vi "Generate symbol map.vi"(11 "M":i32) -> (3 "symbol map":cdb[](array[numeric]) format="%.3f")   [LabVIEW 2011]
uses:
  <vilib>/Analysis/Matrix/Numeric/Conversions/Array To Matrix - RA2.vi
  <vilib>/addons/Modulation/Digital/General/MT Generate Symbol Map (Rectangular).vi
  <vilib>/addons/Modulation/niDMT.lvlib
  <vilib>/Analysis/Matrix/NI_Matrix.lvlib
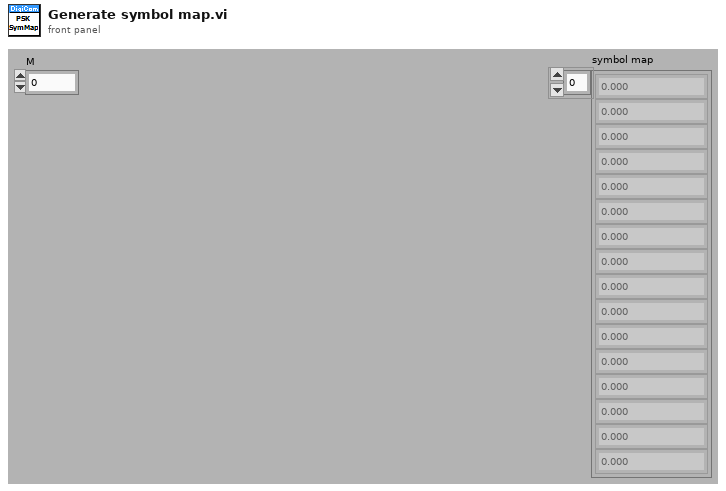
[diagram p1: front panel]
types:
  T1 = typedef "NI_Matrix.lvlib/RealMatrix.ctl" = dbl[][]
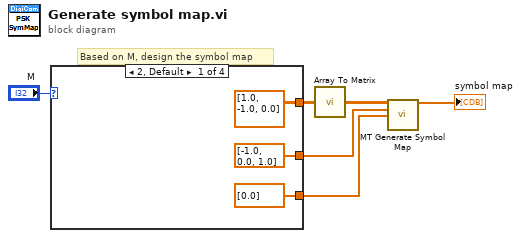
[diagram p0: block diagram]
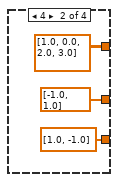
[diagram p2: hidden frame]
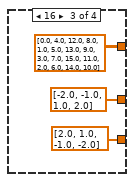
[diagram p3: hidden frame]
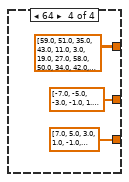
[diagram p4: hidden frame]
diagram:
  # "Based on M, design the symbol map"
  n1 = case shown="2, Default" "M" {
    tunnel: [dbl[][] [[1.0, -1.0, 0.0]] dbl[][] [[1.0, 0.0], [2.0, 3.0]] dbl[][] [[0.0, 4.0, 12.0, 8.0], [1.0, 5.0, 13.0, 9.0], [3.0, 7.0, 15.0, 11.0], [2.0, 6.0, 14.0, 10.0]] dbl[][] [[59.0, 51.0, 35.0, 43.0, 11.0, 3.0, 19.0, 27.0], [58.0, 50.0, 34.0, 42.0, 10.0, 2.0, 18.0, 26.0], [56.0, 48.0, 32.0, 40.0, 8.0, 0.0, 16.0, 24.0], [57.0, 49.0, 33.0, 41.0, 9.0, 1.0, 17.0, 25.0], [61.0, 53.0, 37.0, 45.0, 13.0, 5.0, 21.0, 29.0], [60.0, 52.0, 36.0, 44.0, 12.0, 4.0, 20.0, 28.0], [62.0, 54.0, 38.0, 46.0, 14.0, 6.0, 22.0, 30.0], [63.0, 55.0, 39.0, 47.0, 15.0, 7.0, 23.0, 31.0]]] -> w4
    tunnel: [dbl[] [-1.0, 0.0, 1.0] dbl[] [-1.0, 1.0] dbl[] [-2.0, -1.0, 1.0, 2.0] dbl[] [-7.0, -5.0, -3.0, -1.0, 1.0, 3.0, 5.0, 7.0]] -> w3
    tunnel: [dbl[] [0.0] dbl[] [1.0, -1.0] dbl[] [2.0, 1.0, -1.0, -2.0] dbl[] [7.0, 5.0, 3.0, 1.0, -1.0, -3.0, -5.0, -7.0]] -> w2
    frame 2, Default {
    }
    frame 4 {
    }
    frame 16 {
    }
    frame 64 {
    }
  }
  n2 = call-poly <vilib>:"Array To Matrix.vi"("Real 2D Array"=w4) -> ("Real Matrix"=w1:T1)
  n3 = call-poly <vilib>:"MT Generate Symbol Map.vi"("symbol values"=w1, "symbol amplitudes (I)"=w3, "symbol amplitudes (Q)"=w2) -> ("symbol map"=→"symbol map":cdb[])  [unwired: 11 in, 1 out]
